vi "x410_test_fpga.vi"() -> ()   [LabVIEW 2025]
uses:
  Aqc_loop_states.ctl
  <vilib>/Platform/TimedLoop/XDataNode/timing_clust.ctl
  <vilib>/Platform/TimedLoop/XDataNode/nitl_modes.ctl
  <vilib>/Platform/TimedLoop/XDataNode/wakeup.ctl
  <vilib>/rvi/Emulation/niFpgaSctlEmulationGetInTimedLoop.vi
  <vilib>/rvi/Emulation/niFpgaEmulationReportErrorSimple.vi
  <vilib>/rvi/Emulation/niFpgaGetClockAttributes.vi
  <vilib>/rvi/Emulation/niFpgaCriticalErrorInLSC.vi
  <vilib>/rvi/Emulation/niFpgaProcessEmulError.vi
  <vilib>/rvi/interface/RandomDataEmulation/nirviRandomDataMultiElementFPGAFIFO.vi
  <instcachedir>/0/nirviRandomDataMultiElementFPGAFIFO_BE2FF10D3D6E420AB0291A02835C249E.lvgen/nirviRandomDataMultiElementFPGAFIFO_BE2FF10D3D6E420AB0291A02835C249E_001.vi
  <vilib>/rvi/interface/RandomDataEmulation/niFpgaRandomDataHandleErrors.vi
  <vilib>/Platform/TimedLoop/XDataNode/XDataNode.xnode
  <vilib>/rvi/DataTransferAndStorage/Container/XNode/niFpgaContainer.xnode
  <vilib>/rvi/interface/RandomDataEmulation/nirviRandomDataFpgaMultiElementTemplate.vi
  <vilib>/Platform/TimedLoop/XDataNode/XDNodeRunTimeDep.lvlib
panel:
  in  "Record length":u16=4000 caption="Samples Per Trigger" min=1 step=1
  in  "Trigger Acquisition":bool
  out "loop states":T1
  in  "Acquisition running":bool
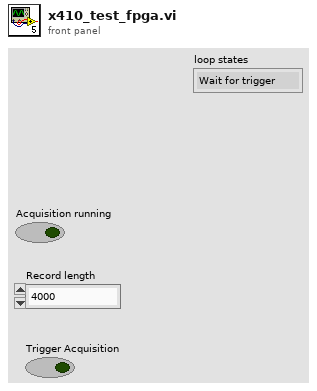
[diagram p1: front panel]
types:
  T1 = typedef "Aqc_loop_states.ctl" = enum8{"Wait for trigger", "Acquisition", "Send record length", "Wait for output", "Quiet period"}
  T2 = typedef "XDNodeRunTimeDep.lvlib/timing_clust.ctl" = cluster{"Expected End [f-1]":u64, "Actual End [f-1]":u64, "Finished Late? [f-1]":bool, "Expected End [i-1]":u64, "Actual End [i-1]":u64, "Finished Late? [i-1]":bool, "Expected Start [i]":u64, "Actual Start [i]":u64, "Expected Start [f]":u64, "Actual Start [f]":u64, "Source Name":string, "Structure Name":string, "Period":i64, "Deadline":i64, "Offset":i64, "Start":i64, "Priority":i32, "Timeout":i32, "Mode":T3, "Wakeup Reason":T4, "Error":errorcluster, "Source Type":string, "Secondary Source Type":string, "Global End Time":u64, "Global Start Time":u64, "Frame Duration":u64, "Iteration Duration":u64, "Assigned CPU":i32, "I/O Scan Engine Mode":u32}
  T3 = typedef "XDNodeRunTimeDep.lvlib/nitl_modes.ctl" = enum32{"No Change", "Process missed periods, maintain original phase", "Discard missed periods, maintain original phase", "Process missed periods, ignore original phase", "Discard missed periods, ignore original phase"}
  T4 = typedef "XDNodeRunTimeDep.lvlib/wakeup.ctl" = enum32{"Normal", "Aborted", "Asynchronous wakeup", "Timing source error", "Timed loop error", "Timeout"}
  T5 = typedef "niInstr DSP v1 Shared.lvlib/IQ Data.ctl" = cluster{"I":fxp<+/-,18,1>, "Q":fxp<+/-,18,1>, "overflow":bool}
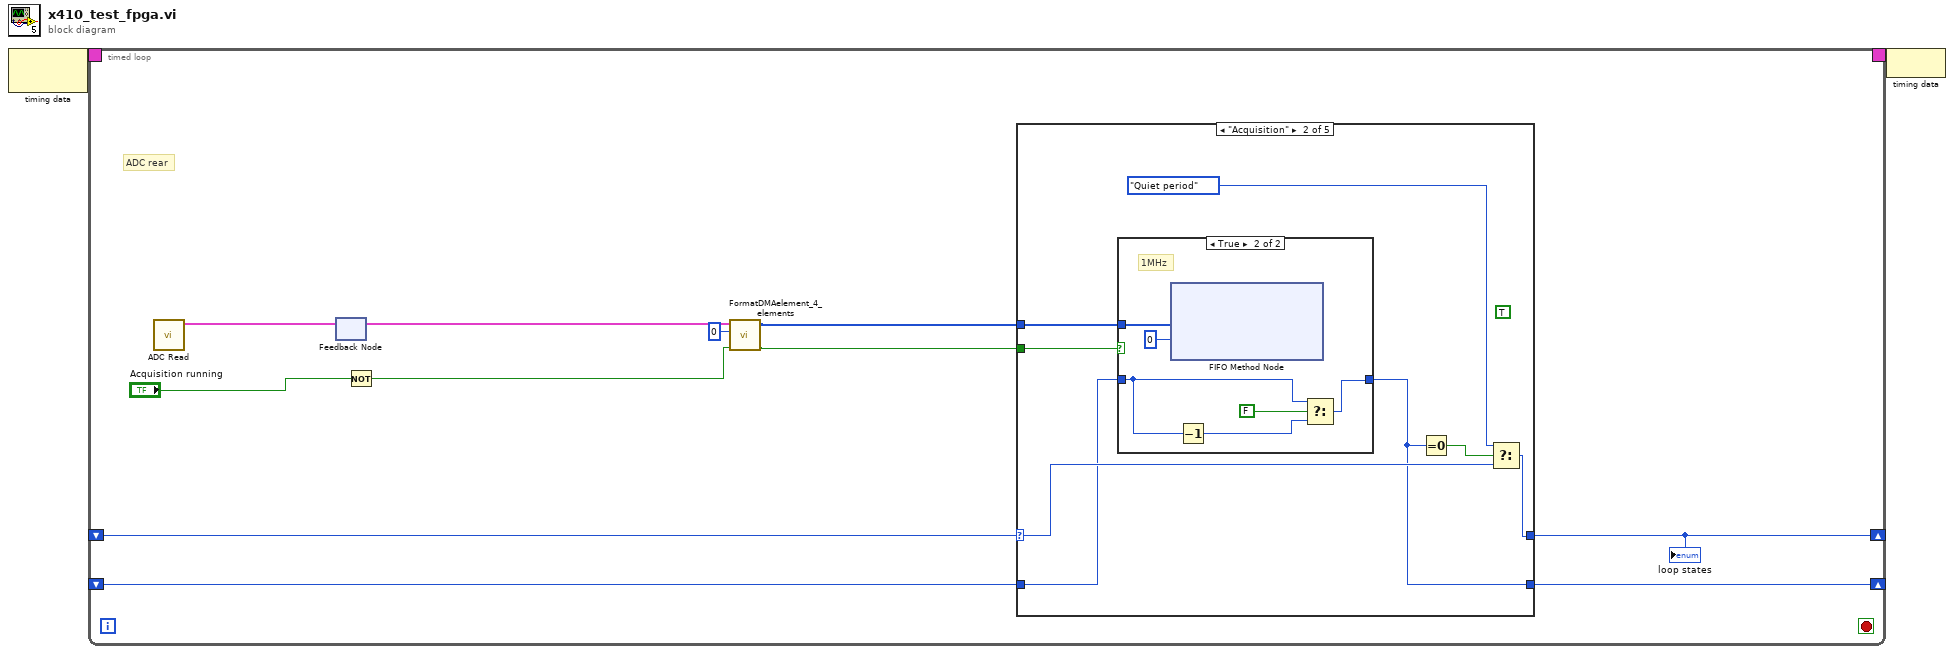
[diagram p0: block diagram]
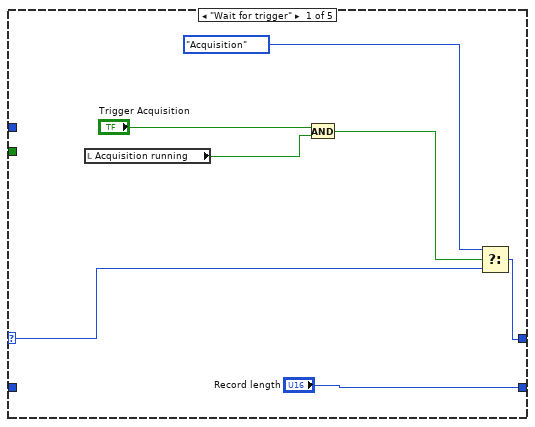
[diagram p2: hidden frame]
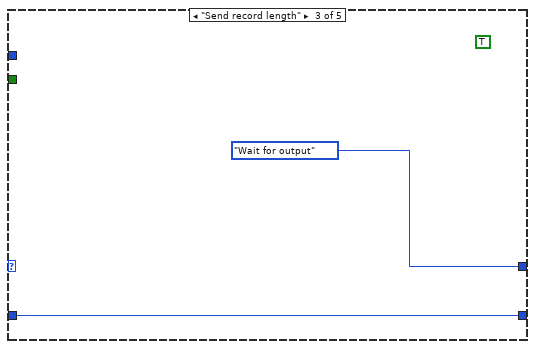
[diagram p4: hidden frame]
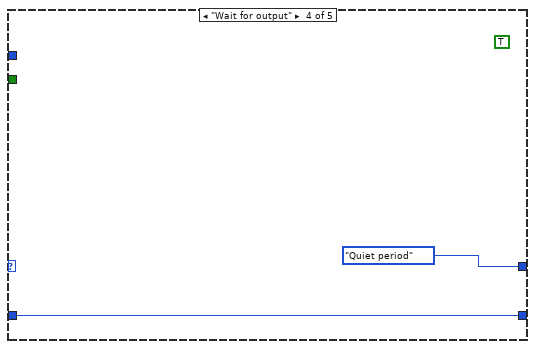
[diagram p5: hidden frame]
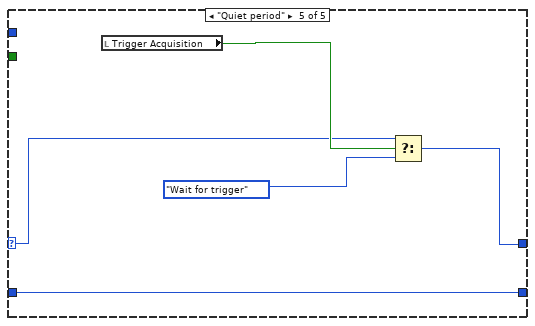
[diagram p6: hidden frame]
diagram:
  n1 = node-c288() -> (w2:T2)  [unwired: 1 in]
  n2 = timed-loop {
    timing: w2 -> [_]
    timing-out: [_] -> w1
    shift-right: [w11] -> _
    shift-left: _ -> [w13]
    shift-right: [w10] -> _
    shift-left: _ -> [w12]
    stop <- _ stop-if-true
    # "ADC rear"
    n3 = call "ADC Read.vi"() -> ("Data out"=w8:T5[])  [unwired: 11 in]
    n4 = feedback #1() -> (w7:T5[])  [unwired: 1 in]
    n5 = feedback-in #1(w8) -> ()
    n6 = Not(x="Acquisition running") -> (.not. x?=w6:bool)
    n7 = call "FormatDMAelement_4_elements.vi"("valid in"=w6, "factor"=u16 0, "Data int"=w7) -> ("valid out"=w5:bool, "Values"=w4:u64[])  [unwired: 7 in]
    n8 = case shown="\"Acquisition\"" w13 {
      selector: w13 -> [w20 w28 _ _ w41]
      tunnel: w12 -> [_ w25 w37 w39 w42]
      tunnel: [w19 w27 Aqc_loop_states."Wait for output" ("loop states") Aqc_loop_states."Quiet period" ("loop states") w43] -> w11
      tunnel: ["Record length" w22 w37 w39 w42] -> w10
      tunnel: w4 -> [_ w23 _ _ _]
      tunnel: w5 -> [_ w24 _ _ _]
      frame "Wait for trigger" {
        n9 = local read "Acquisition running"() -> (w18:bool)
        n10 = And(x="Trigger Acquisition", y=w18) -> (x .and. y?=w16:bool)
        n11 = Select(t=Aqc_loop_states."Acquisition" ("loop states"), s=w16, f=w20) -> (s? t:f=w19:T1)
      }
      frame "Acquisition" {
        (unwired) TRUE
        n12 = case shown="True" w24 {
          tunnel: w23 -> [_ w35]
          tunnel: [w29 w33] -> w22
          tunnel: w25 -> [w29 w31]
          frame False {
          }
          frame True {
            # "1MHz"
            n13 = xnode ("FIFO Method Node")("Element"=w35, "Timeout"=0) -> ()  [unwired: 1 in, 2 out]
            n14 = Decrement(x=w31) -> (x-1=w32:u16)
            n15 = Select(t=w31, s=FALSE, f=w32) -> (s? t:f=w33:u16)
          }
        }
        n16 = Equal To 0?(x=w22) -> (x = 0?=w26:bool)
        n17 = Select(t=Aqc_loop_states."Quiet period" ("loop states"), s=w26, f=w28) -> (s? t:f=w27:T1)
      }
      frame "Send record length" {
        (unwired) TRUE ("5782 triggered")
      }
      frame "Wait for output" {
        (unwired) TRUE ("5782 triggered")
      }
      frame "Quiet period" {
        n18 = local read "Trigger Acquisition"() -> (w44:bool)
        n19 = Select(t=w41, s=w44, f=Aqc_loop_states."Wait for trigger" ("loop states")) -> (s? t:f=w43:T1)
      }
    }
    "loop states" <- w11
  }
  n20 = node-c288(w1) -> ()
